vi "采集数字.vi"() -> ()   [LabVIEW 2018]
panel:
  out "F-格式字符串":string
  in  "布尔 2":bool
  out "波形图表":dbl(graph)
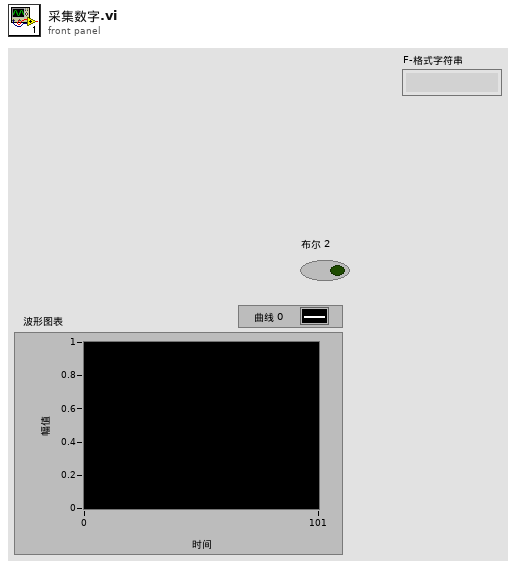
[diagram p1: front panel]
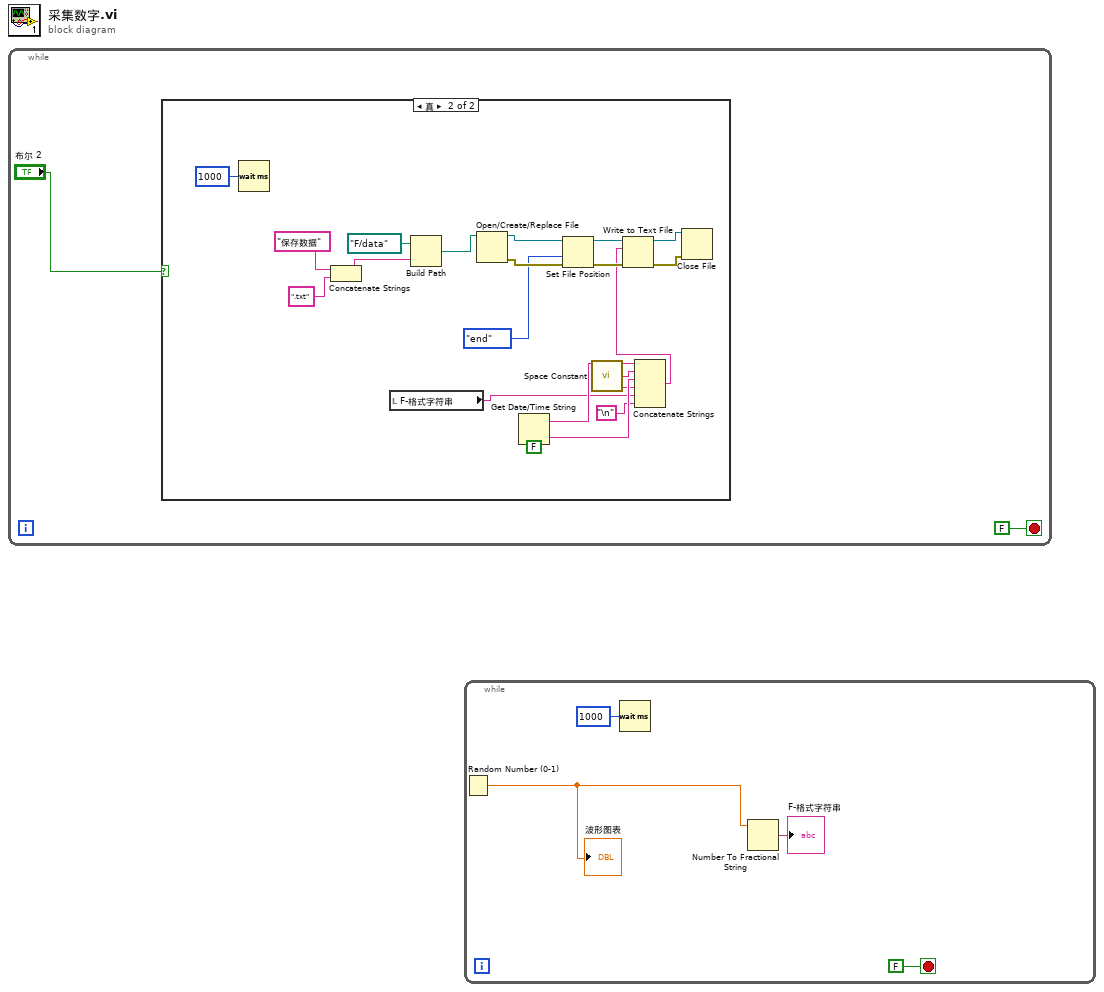
[diagram p0: block diagram]
diagram:
  n1 = while {
    stop <- FALSE stop-if-true
    n2 = case shown="真" "布尔 2" {
      frame False {
      }
      frame True {
        n3 = Wait (ms)(milliseconds to wait=u32 1000 ("等待时间（毫秒）")) -> ()  [unwired: 1 out]
        n4 = Concatenate Strings("保存数据", ".txt") -> (w20:string)
        n5 = local read "F-格式字符串"() -> (w4:string)
        n6 = Build Path(base path=path "F:/data" ("基路径"), name or relative path=w20) -> (appended path=w19:path)
        n7 = Open/Create/Replace File(file path (use dialog)=w19) -> (refnum out=w18:refnum<file>, error out=w17:errorcluster)  [unwired: 5 in, 1 out]
        n8 = Get Date/Time String(want seconds? (F)=FALSE ("需要秒？(F)")) -> (date string=w9:string, time string=w7:string)  [unwired: 2 in]
        n9 = Set File Position(refnum=w18, from (0:start)=enum16{"start", "end", "current"}."end" ("自（0:起始）"), error in=w17) -> (refnum out=w16:refnum<file>, error out=w15:errorcluster)  [unwired: 1 in]
        n10 = call <vilib>:"Space Constant.vi"() -> ("String"=w6:string)
        n11 = Concatenate Strings(w9, w6, w7, w6, w4, "\n") -> (w8:string)
        n12 = Write to Text File(file (use dialog)=w16, text=w8, error in=w15) -> (refnum out=w14:refnum<file>, error out=w13:errorcluster)  [unwired: 1 in, 1 out]
        n13 = Close File(refnum=w14, error in=w13) -> ()  [unwired: 2 out]
      }
    }
  }
  n14 = while {
    stop <- FALSE stop-if-true
    n15 = Random Number (0-1)() -> (number: 0 to 1=w24:dbl)
    "波形图表" <- w24
    n16 = Wait (ms)(milliseconds to wait=u32 1000 ("等待时间（毫秒）")) -> ()  [unwired: 1 out]
    n17 = Number To Fractional String(number=w24) -> (F-format string=→"F-格式字符串":string)  [unwired: 3 in]
  }
